vi "GoForward.vi"(0 "reference in":refnum<class "DP_WebView.lvclass">, 5 "Error In":errorcluster) -> (14 "reference out":refnum<class "DP_WebView.lvclass">, 19 "Error Out":errorcluster)   [LabVIEW 2020, in "DP_WebView.lvclass"]
uses:
  DP_WebView.lvclass
  C:/Projects/DependencyViewer/DependencyViewer/DP_WebView_class/data/Microsoft.Web.WebView2.Core.dll
  data/Microsoft.Web.WebView2.Core.dll
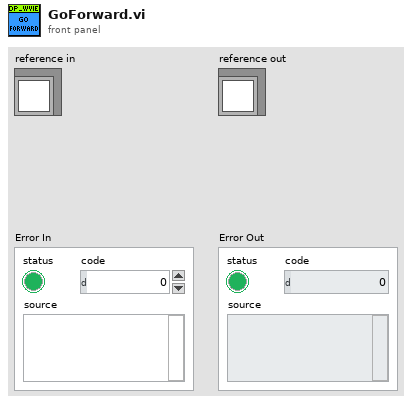
[diagram p1: front panel]
types:
  T1 = typedef "DP_WebView.lvclass/ObjectAttributes.ctl" = cluster{"WebView Container":refnum<k24>, "CoreWebViewRef":refnum<k24>, "Status":i32, "Status Message":string, "User Data Folder":path, "BrowserProcessId":u32}
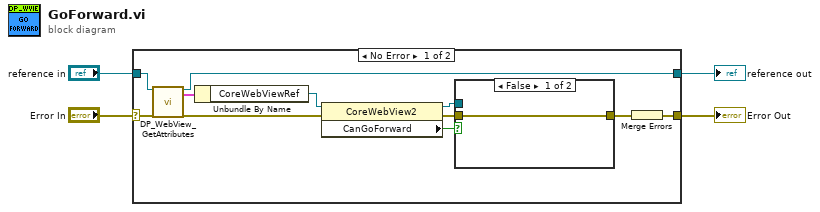
[diagram p0: block diagram]
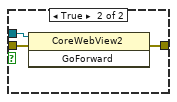
[diagram p2: hidden frame]
diagram:
  n1 = case shown="No Error" "Error In" {
    selector: "Error In" -> [w15 w21]
    tunnel: [w12 w21] -> w3
    tunnel: [w13 w20] -> w1
    tunnel: "reference in" -> [w14 w20]
    frame No Error {
      n2 = call "DP_WebView_GetAttributes.vi"("reference in"=w14, "error in (no error)"=w15) -> ("reference out"=w13:refnum<class "DP_WebView.lvclass">, "Data"=w11:T1, "error out"=w5:errorcluster)  [unwired: 14 in, 1 out]
      n3 = Unbundle By Name(w11) -> ("CoreWebViewRef"=w9:refnum<k24>)
      n4 = property class="CoreWebView2"(reference=w9, error in=w5) -> (reference out=w8:refnum<k24>, error out=w6:errorcluster, "CanGoForward"=w7:bool)
      n5 = case shown="False" w7 {
        tunnel: w6 -> [w16 w19]
        tunnel: [w16 w18] -> w10
        tunnel: w8 -> [_ w17]
        frame False {
        }
        frame True {
          n6 = invoke class="CoreWebView2" method="GoForward"(reference=w17, error in=w19) -> (error out=w18:errorcluster)  [unwired: 1 in, 2 out]
        }
      }
      n7 = Merge Errors(w10) -> (w12:errorcluster)
    }
    frame Error {
    }
  }
  "Error Out" <- w3
  "reference out" <- w1
